vi "Water Tank 1.vi"() -> ()   [LabVIEW 2024]
panel:
  in  "stop":bool
  out "Tank":dbl(slide) scale=0.0..100.0
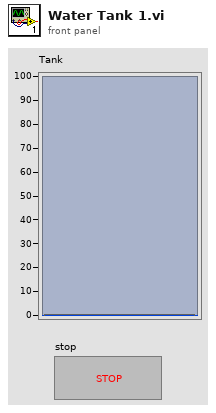
[diagram p1: front panel]
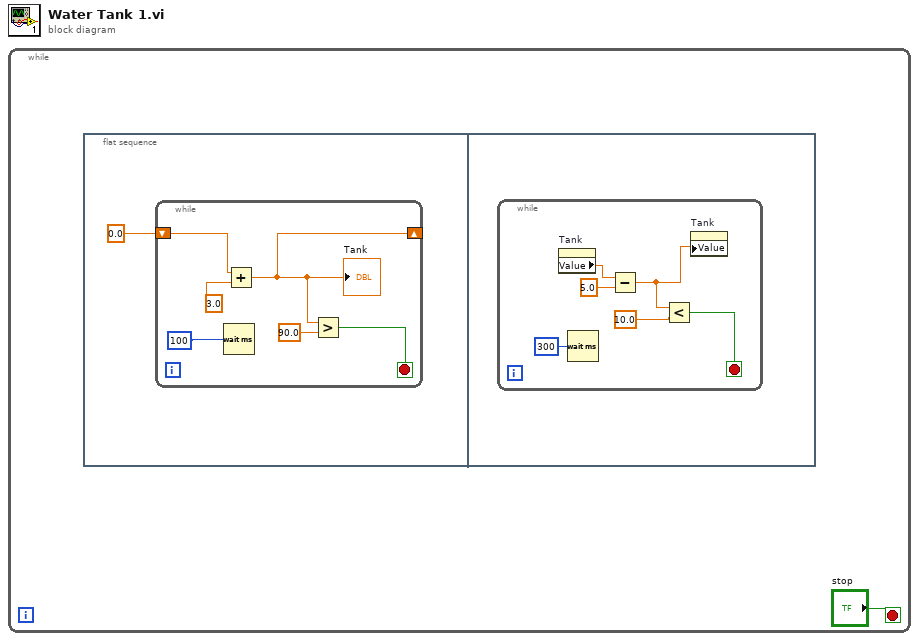
[diagram p0: block diagram]
diagram:
  n1 = while {
    stop <- "stop" stop-if-true
    n2 = flat-sequence {
      frame #0 {
        n3 = while {
          shift-right: [w5] -> _
          shift-left: 0.0 -> [w8]
          stop <- w3 stop-if-true
          n4 = Wait (ms)(milliseconds to wait=u32 100 ("millisecond timer value")) -> ()  [unwired: 1 out]
          n5 = Add(x=w8, y=3.0) -> (x+y=w5:dbl)
          "Tank" <- w5
          n6 = Greater?(x=w5, y=90.0) -> (0:w3:bool)
        }
      }
      frame #1 {
        n7 = while {
          stop <- w10 stop-if-true
          n8 = property on="Tank" class="Slide (strict)"() -> ("Value"=w14:dbl)  [unwired: 2 in, 2 out]
          n9 = Wait (ms)(milliseconds to wait=u32 300) -> ()  [unwired: 1 out]
          n10 = Subtract(x=w14, y=5.0) -> (x-y=w12:dbl)
          n11 = Less?(x=w12, y=10.0) -> (x < y?=w10:bool)
          n12 = property on="Tank" class="Slide (strict)"("Value"=w12) -> ()  [unwired: 2 in, 2 out]
        }
      }
    }
  }
